vi "Request.vi"(0 "object in":refnum<class "ITarget.lvclass">, 5 "Data":T1, 11 "Error In":errorcluster) -> (4 "object out":refnum<class "ITarget.lvclass">, 15 "Error Out":errorcluster)   [LabVIEW 2024, in "ITarget.lvclass"]
uses:
  ITarget.lvclass
  Support/SignalData.ctl
panel:
  # "Connector Pane"
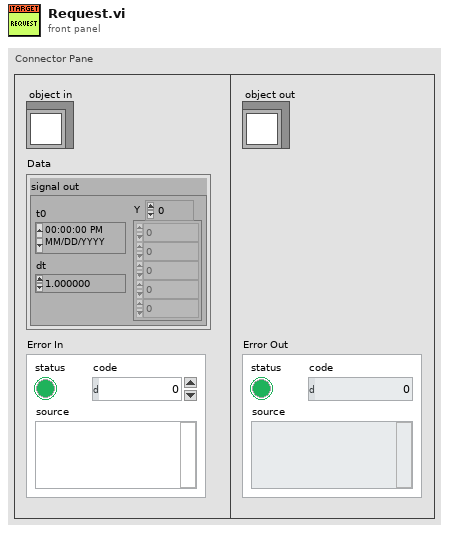
[diagram p1: front panel]
types:
  T1 = typedef "SignalData.ctl" = cluster{"signal out":waveform(dbl)}
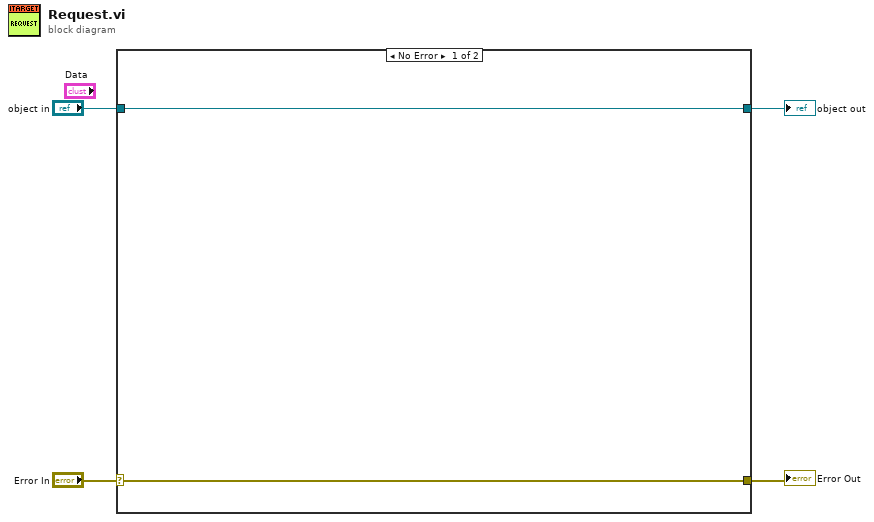
[diagram p0: block diagram]
diagram:
  n1 = case shown="No Error" "Error In" {
    selector: "Error In" -> [w6 w8]
    tunnel: [w6 w8] -> w3
    tunnel: [w5 w7] -> w1
    tunnel: "object in" -> [w5 w7]
    frame No Error {
    }
    frame Error {
    }
  }
  "Error Out" <- w3
  "object out" <- w1
